vi "MainRIO_1.vi"() -> ()   [LabVIEW 2013]
uses:
  <vilib>/Platform/TimedLoop/XDataNode/timing_clust.ctl
  <vilib>/Platform/TimedLoop/XDataNode/nitl_modes.ctl
  <vilib>/Platform/TimedLoop/XDataNode/wakeup.ctl
  <vilib>/myRIO/Instrument Drivers/Onboard IO/AO/vis/Smart Open.vi
  <vilib>/myRIO/Instrument Drivers/Onboard IO/AO/vis/Write.vi
  <vilib>/myRIO/Instrument Drivers/Onboard IO/AO/vis/Open.vi
  <vilib>/myRIO/Common/Instrument Driver Framework/myRIO v1.0/AO/vis/myRIO v1.1 Open AO.vi
  <vilib>/myRIO/Common/Instrument Driver Framework/Utilities/vis/Validate Channels.vi
  <vilib>/myRIO/Common/Instrument Driver Framework/myRIO v1.0/AO/vis/myRIO v1.0 Reserve AO.vi
  <vilib>/myRIO/Common/Instrument Driver Framework/myRIO v1.0/AO/vis/myRIO v1.0 Build MUX Configuration AO.vi
  <vilib>/myRIO/Common/Instrument Driver Framework/myRIO v1.0/Resource Manager/vis/myRIO v1.0 Reserve Channel List.vi
  <vilib>/myRIO/Common/Instrument Driver Framework/myRIO v1.0/Resource Manager/vis/myRIO v1.0 Reserve Channel.vi
  <vilib>/myRIO/Common/Instrument Driver Framework/myRIO v1.0/Resource Manager/vis/myRIO v1.0 Unreserve Channel.vi
  <vilib>/myRIO/Common/Instrument Driver Framework/myRIO v1.0/Resource Manager/vis/myRIO v1.0 Build Mutex Name.vi
  <vilib>/myRIO/Common/Instrument Driver Framework/myRIO v1.0/myRIO v1.1 Open.vi
  <vilib>/myRIO/Common/Instrument Driver Framework/myRIO v1.0/AO/vis/myRIO v1.0 Get Scaling Constants AO.vi
  <vilib>/Utility/VariantDataType/GetNumericInfo.vi
  <vilib>/Utility/error.llb/Error Cluster From Error Code.vi
  <vilib>/myRIO/Common/Instrument Driver Framework/Utilities/vis/IO Manager.vi
  <vilib>/myRIO/Common/Instrument Driver Framework/Utilities/vis/Configuration Manager.vi
  <vilib>/myRIO/Common/Instrument Driver Framework/myRIO v1.0/myRIO v1.0 Close.vi
  <vilib>/myRIO/Common/Instrument Driver Framework/myRIO v1.0/AO/vis/myRIO v1.0 Write AO.vi
  <vilib>/platform/TimedLoop/XDataNode/XDataNode.xnode
  <vilib>/Platform/TimedLoop/XDataNode/XDNodeRunTimeDep.lvlib
panel:
  out "Velocity Voltage without limit (not sent to RIO)":dbl
  out "VelocityReference to Controller":dbl
  out "RIOparameters_1":T1
  out "Velocoty Voltage (Uy)":dbl=2.1
  out "Steering Voltage (Ux)":dbl=2.0
  in  "PID gains Velocity control":T2={"proportional gain (Kc)"=1.0, "integral time (Ti, min)"=0.01, "derivative time (Td, min)"=0.0} {"derivative time (Td, min)" step=0.01 format="%.3f"; "integral time (Ti, min)" format="%.3f"; "proportional gain (Kc)" step=0.05 format="%.3f"}
  in  "PID gains PathController":T2={"proportional gain (Kc)"=600.0, "integral time (Ti, min)"=0.25, "derivative time (Td, min)"=0.01} {"derivative time (Td, min)" format="%.3f"; "integral time (Ti, min)" format="%.3f"; "proportional gain (Kc)" format="%.3f"}
  in  "Proportional constant DistanceError":dbl=0.4 step=0.1
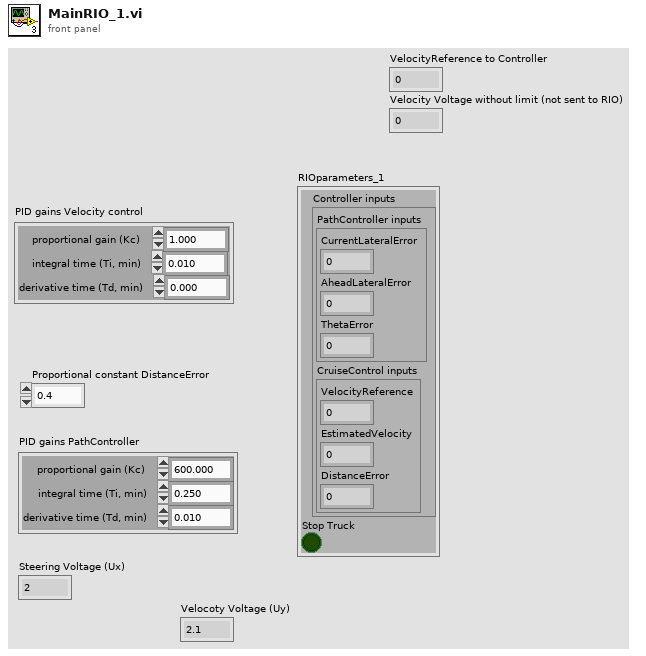
[diagram p1: front panel]
types:
  T1 = cluster{"Controller inputs":cluster{"PathController inputs":cluster{"CurrentLateralError":dbl, "AheadLateralError":dbl, "ThetaError":dbl}, "CruiseControl inputs":cluster{"VelocityReference":dbl, "EstimatedVelocity":cdb, "DistanceError":cdb}}, "Stop Truck":bool}
  T2 = cluster{"proportional gain (Kc)":dbl, "integral time (Ti, min)":dbl, "derivative time (Td, min)":dbl}
  T3 = typedef "XDNodeRunTimeDep.lvlib/timing_clust.ctl" = cluster{"Expected End [f-1]":u64, "Actual End [f-1]":u64, "Finished Late? [f-1]":bool, "Expected End [i-1]":u64, "Actual End [i-1]":u64, "Finished Late? [i-1]":bool, "Expected Start [i]":u64, "Actual Start [i]":u64, "Expected Start [f]":u64, "Actual Start [f]":u64, "Source Name":string, "Structure Name":string, "Period":i64, "Deadline":i64, "Offset":i64, "Start":i64, "Priority":i32, "Timeout":i32, "Mode":T4, "Wakeup Reason":T5, "Error":errorcluster, "Source Type":string, "Secondary Source Type":string, "Global End Time":u64, "Global Start Time":u64, "Frame Duration":u64, "Iteration Duration":u64, "Assigned CPU":i32, "I/O Scan Engine Mode":u32}
  T4 = typedef "XDNodeRunTimeDep.lvlib/nitl_modes.ctl" = enum32{"No Change", "Process missed periods, maintain original phase", "Discard missed periods, maintain original phase", "Process missed periods, ignore original phase", "Discard missed periods, ignore original phase"}
  T5 = typedef "XDNodeRunTimeDep.lvlib/wakeup.ctl" = enum32{"Normal", "Aborted", "Asynchronous wakeup", "Timing source error", "Timed loop error", "Timeout"}
  T6 = cluster{"CurrentLateralError":dbl, "AheadLateralError":dbl, "ThetaError":dbl}
  T7 = cluster{"VelocityReference":dbl, "EstimatedVelocity":cdb, "DistanceError":cdb}
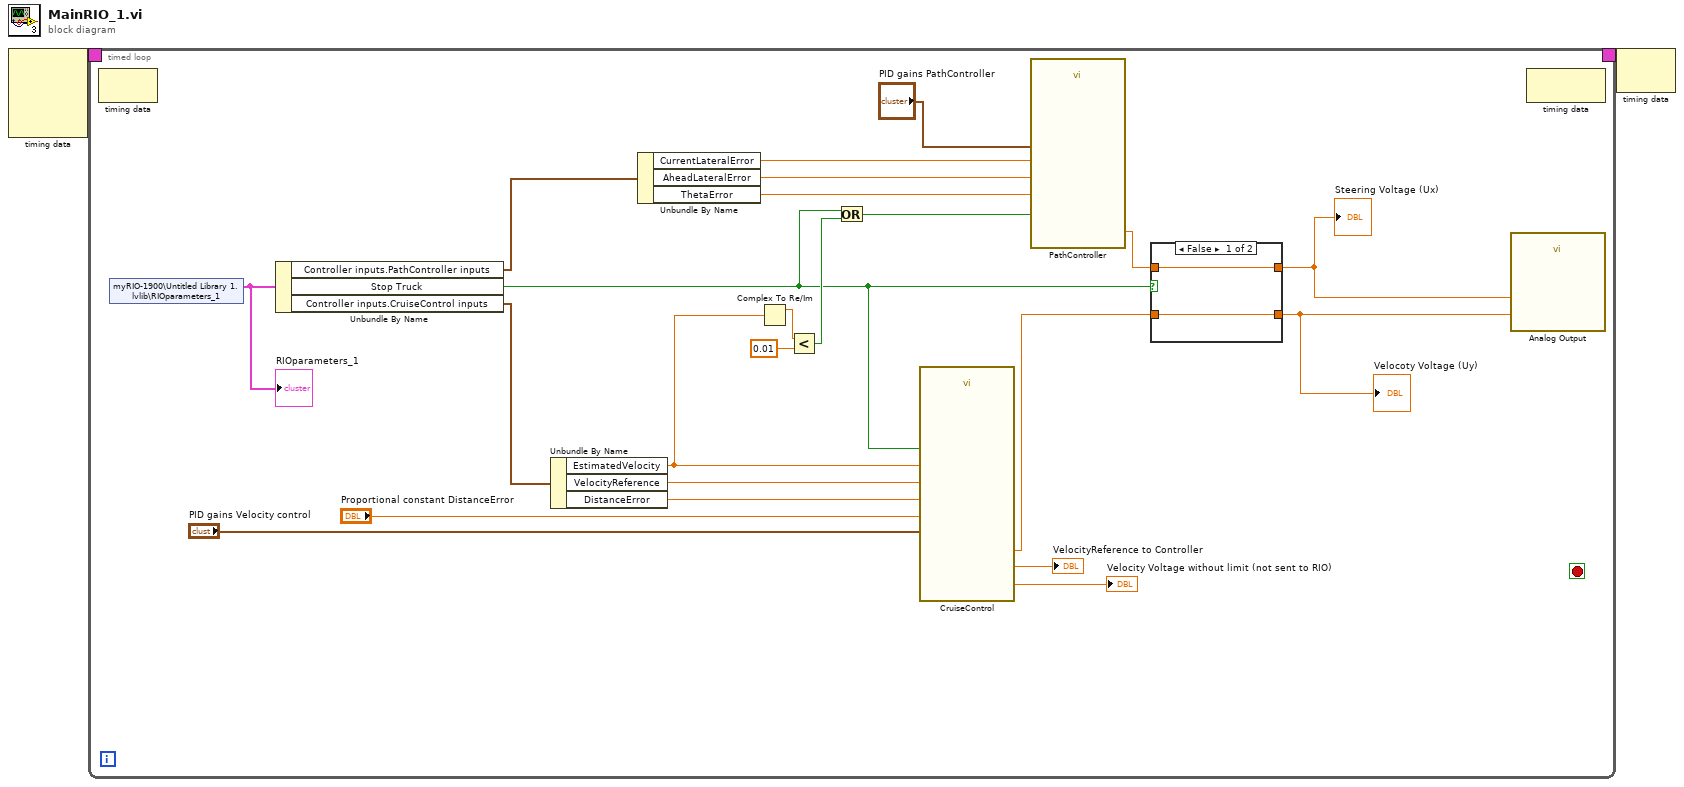
[diagram p0: block diagram]
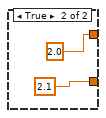
[diagram p2: hidden frame]
diagram:
  n1 = node-c288() -> (w2:T3)  [unwired: 4 in]
  n2 = timed-loop {
    timing: w2 -> [_]
    timing-out: [_] -> w1
    stop <- _ stop-if-true
    n3 = node-c288() -> ()  [unwired: 1 in, 1 out]
    n4 = shared-variable "myRIO-1900\\Untitled Library 1.lvlib\\RIOparameters_1"() -> (w19:T1)  [unwired: 1 in, 1 out]
    "RIOparameters_1" <- w19
    n5 = Unbundle By Name(w19) -> ("Controller inputs.PathController inputs"=w21:T6, "Stop Truck"=w10:bool, "Controller inputs.CruiseControl inputs"=w20:T7)
    n6 = Unbundle By Name(w20) -> ("EstimatedVelocity"=w15:cdb, "VelocityReference"=w14:dbl, "DistanceError"=w13:cdb)
    n7 = Unbundle By Name(w21) -> ("CurrentLateralError"=w7:dbl, "AheadLateralError"=w6:dbl, "ThetaError"=w5:dbl)
    n8 = Complex To Re/Im(x + iy=w15) -> (x=w23:dbl)  [unwired: 1 out]
    n9 = Less?(x=w23, y=0.01) -> (x < y?=w16:bool)
    n10 = Or(x=w10, y=w16) -> (x .or. y?=w9:bool)
    n11 = call "CruiseControl.vi"("reinitialize? (F)"=w10, "PID gains Velocity control"="PID gains Velocity control", "DistanceError"=w13, "EstimatedVelocity"=w15, "VelocityReference"=w14, "K"="Proportional constant DistanceError") -> ("VelocityReference to Controller"=→"VelocityReference to Controller":dbl, "Velocity Voltage without limit (not sent to RIO)"=→"Velocity Voltage without limit (not sent to RIO)":dbl, "Velocity Voltage"=w17:dbl)  [unwired: 3 in]
    n12 = call "PathController.vi"("PID gains"="PID gains PathController", "reinitialize? (F)"=w9, "ThetaError"=w5, "AheadLateralError"=w6, "CurrentLateralError"=w7) -> ("Steering Voltage"=w4:dbl)  [unwired: 6 in]
    n13 = case shown="False" w10 {
      tunnel: [w26 2.0 ("Steering Voltage")] -> w25
      tunnel: [w27 2.1 ("Uy")] -> w24
      tunnel: w17 -> [w27 _]
      tunnel: w4 -> [w26 _]
      frame False {
      }
      frame True {
      }
    }
    "Velocoty Voltage (Uy)" <- w24
    "Steering Voltage (Ux)" <- w25
    n14 = call "Analog Output"("C/AO0"=w25, "C/AO1"=w24) -> ()  [unwired: 25 in, 1 out]
    n15 = node-c288() -> ()  [unwired: 1 in, 1 out]
  }
  n16 = node-c288(w1) -> ()  [unwired: 1 out]
